vi "Copy Text To Clipboard.vi"(1 "Text to copy to clipboard":string) -> (0 "Error Out":cluster{bool, i32, "source":string})   [LabVIEW 8.6]
doc: "copys text to the Windows clipboard\n\n2002 by Arnold Bartel"
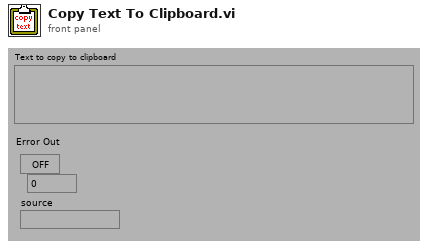
[diagram p1: front panel]
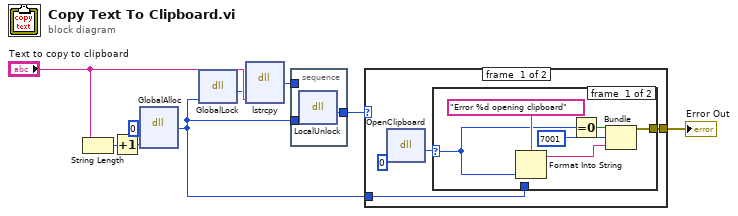
[diagram p0: block diagram]
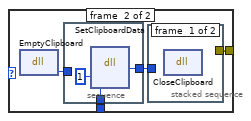
[diagram p2: hidden frame]
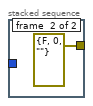
[diagram p3: hidden frame]
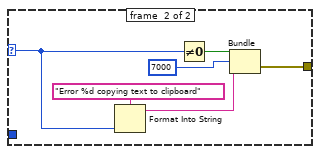
[diagram p4: hidden frame]
diagram:
  n1 = String Length(string="Text to copy to clipboard") -> (length=w8:i32)
  n2 = Increment(x=w8) -> (x+1=w4:i32)
  n3 = dll-call lib="kernel32" fn="GlobalAlloc"("Flags"=i16 0 ("Format"), "Size"=w4) -> (w3:i32)  [unwired: 5 in, 2 out]
  n4 = dll-call lib="kernel32" fn="GlobalLock"("hGlobalMemory"=w3) -> (w6:i32)  [unwired: 4 in, 2 out]
  n5 = dll-call lib="kernel32" fn="lstrcpy"("Flags"=w6, "String"="Text to copy to clipboard") -> (w5:i32)  [unwired: 5 in, 2 out]
  n6 = stacked-sequence {
    tunnel: w5 -> [_]
    tunnel: w3 -> [w11]
    tunnel: [w10] -> w2
    frame #0 {
      n7 = dll-call lib="kernel32" fn="LocalUnlock"("hGlobalMemory"=w11) -> (w10:i32)  [unwired: 4 in, 2 out]
    }
  }
  n8 = case shown="0" w2 {
    selector: w2 -> [_ w32]
    tunnel: w3 -> [w14 _]
    tunnel: [w12 w34] -> w1
    frame #0 {
      n9 = dll-call lib="user32" fn="OpenClipboard"("owner"=i16 0) -> (w13:i32)  [unwired: 4 in, 2 out]
      n10 = case shown="1, Default" w13 {
        selector: w13 -> [w17 _]
        tunnel: w14 -> [_ w24]
        tunnel: [w20 w22] -> w12
        frame #0 {
          n11 = Format Into String(format string="Error %d opening clipboard" ("source"), w17) -> (resulting string=w18:string)  [unwired: 2 in, 1 out]
          n12 = Equal To 0?(x=w17) -> (x = 0?=w21:bool)
          n13 = Bundle(w21, 7001, w18) -> (w20:errorcluster)  [unwired: 1 in]
        }
        frame #1 {
          n14 = dll-call lib="user32" fn="EmptyClipboard"() -> (w25:i32)  [unwired: 3 in, 2 out]
          n15 = stacked-sequence {
            tunnel: w25 -> [_]
            tunnel: w24 -> [w28]
            tunnel: [w27] -> w23
            frame #0 {
              n16 = dll-call lib="user32" fn="SetClipboardData"("Format"=1, "Data"=w28) -> (w27:i32)  [unwired: 5 in, 2 out]
            }
          }
          n17 = stacked-sequence {
            tunnel: w23 -> [_ _]
            tunnel: [_ cluster{bool, i32, "source":string} {FALSE, 0, "source"=""} ("Output Element")] -> w22
            frame #0 {
              n18 = dll-call lib="user32" fn="CloseClipboard"() -> ()  [unwired: 4 in, 2 out]
            }
            frame #1 {
            }
          }
        }
      }
    }
    frame #1 {
      n19 = Format Into String(format string="Error %d copying text to clipboard" ("source"), w32) -> (resulting string=w31:string)  [unwired: 2 in, 1 out]
      n20 = Not Equal To 0?(x=w32) -> (x != 0?=w35:bool)
      n21 = Bundle(w35, 7000, w31) -> (w34:errorcluster)  [unwired: 1 in]
    }
  }
  "Error Out" <- w1
